vi "ServiceSendBytesRoutedMessage_Parse.vi"(8 "error in (no error)":errorcluster, 11 "Message":T5) -> (0 "error out":errorcluster, 1 "Body":T1, 2 "Header":T3, 3 "ServiceSendBytesRoutedMessage":T2)   [LabVIEW 2017]
uses:
  <vilib>/addons/InsightCM/MessageBus/Base/controls/Message.ctl
  <vilib>/addons/InsightCM/MessageBus/Base/controls/MessageHeader.ctl
  <vilib>/addons/InsightCM/MessageBus/Base/controls/KeyValuePair.ctl
  <vilib>/addons/InsightCM/MessageBus/MessageLibrary/Service/controls/ServiceSendBytesRoutedMessage.ctl
  <vilib>/addons/InsightCM/MessageBus/MessageLibrary/Service/controls/ServiceSendBytesRoutedMessageBody.ctl
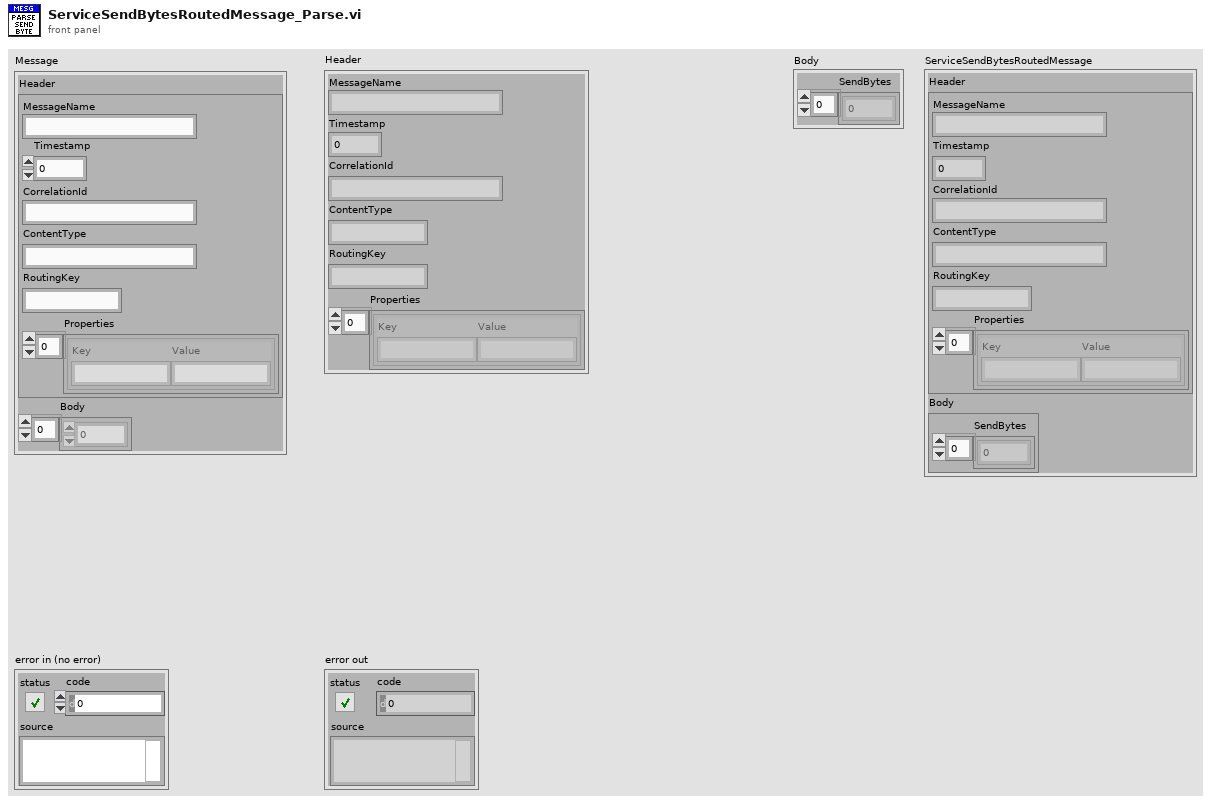
[diagram p1: front panel]
types:
  T1 = typedef "ServiceSendBytesRoutedMessageBody.ctl" = cluster{"SendBytes":u8[]}
  T2 = typedef "ServiceSendBytesRoutedMessage.ctl" = cluster{"Header":T3, "Body":T1}
  T3 = typedef "MessageHeader.ctl" = cluster{"MessageName":string, "Timestamp":i64, "CorrelationId":string, "ContentType":string, "RoutingKey":string, "Properties":T4[]}
  T4 = typedef "KeyValuePair.ctl" = cluster{"Key":string, "Value":string}
  T5 = typedef "Message.ctl" = cluster{"Header":T3, "Body":u8[]}
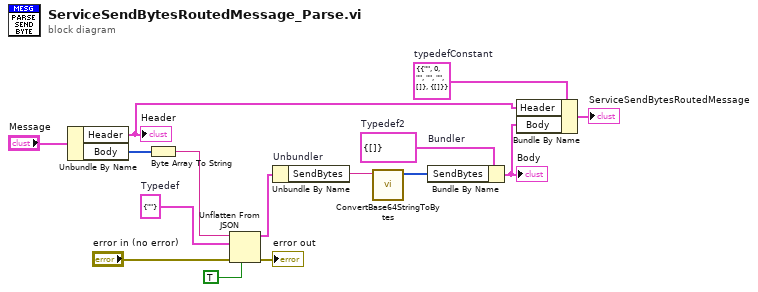
[diagram p0: block diagram]
diagram:
  w3 = T1 {"SendBytes"=[]}  # Typedef2
  w7 = T2 {"Header"={"MessageName"="", "Timestamp"=0, "CorrelationId"="", "ContentType"="", "RoutingKey"="", "Properties"=[]}, "Body"={"SendBytes"=[]}}  # typedefConstant
  w11 = cluster{"SendBytes":string} {"SendBytes"=""}  # Typedef
  n1 = Unbundle By Name("Message") -> ("Header"=w13:T3, "Body"=w5:u8[])
  "Header" <- w13
  n2 = Byte Array To String(unsigned byte array=w5) -> (string=w10:string)
  n3 = Unflatten From JSON(JSON string=w10, type and defaults=w11, default null elements? (F)=TRUE, error in (no error)="error in (no error)") -> (value=w9:cluster{"SendBytes":string}, error out=→"error out":errorcluster)  [unwired: 3 in]
  n4 = Unbundle By Name "Unbundler"(w9) -> ("SendBytes"=w2:string)
  n5 = call <vilib>:"ConvertBase64StringToBytes.vi"("Base64 string"=w2) -> ("U8 array"=w1:u8[])  [unwired: 9 in, 1 out]
  n6 = Bundle By Name "Bundler"(cluster=w3, "SendBytes"=w1) -> (w4:T1)
  "Body" <- w4
  n7 = Bundle By Name(cluster=w7, "Header"=w13, "Body"=w4) -> (→"ServiceSendBytesRoutedMessage":T2)
